vi "Initialize.vi"(7 "Serial Configuration":T1={"Baud Rate"=9600, "Parity"=0, "Data Bits"=8} {"Data Bits" items=["7"=7, "8"=8]; "Parity" items=["None", "Odd", "Even"]; "Baud Rate" items=["300"=300, "600"=600, "1200"=1200, "2400"=2400, "4800"=4800, "9600"=9600]}, 8 "error in (no error)":errorcluster, 9 "Reset (True)":bool=TRUE, 10 "ID Query (True)":bool=TRUE, 11 "VISA resource name":refnum<visa-resource-name>) -> (0 "error out":errorcluster, 3 "VISA resource name out":refnum<visa-resource-name>)   [LabVIEW 2022 SP3, in "Agilent 34420.lvlib"]
doc: "Establishes communication with the instrument and optionally performs an instrument identification query and/or an instrument reset. It also places the instrument in a default state needed for other instrument driver operations. Therefore, call this VI before calling other instrument driver VIs for this instrument. Generally, you need to call the Initialize VI only once at the beginning of an application."
uses:
  Agilent 34420.lvlib
  <vilib>/regexp/Match Regular Expression.xnode
  agilent_n6900_n7900_series/Agilent N6900 N7900 Series/Agilent N6900 N7900 Series.lvlib
panel:
  # "(c) 2008-2015 National Instruments Corp.  ALL RIGHTS RESERVED."
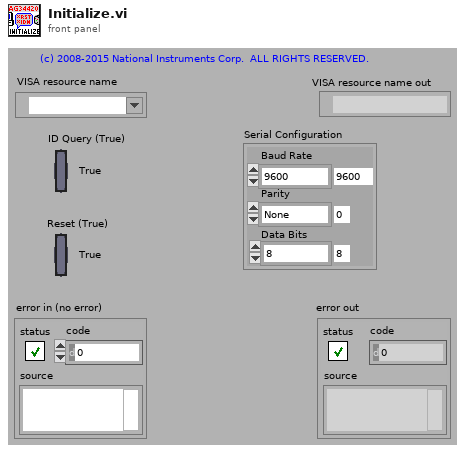
[diagram p1: front panel]
types:
  T1 = cluster{"Baud Rate":u32, "Parity":u16, "Data Bits":u16}
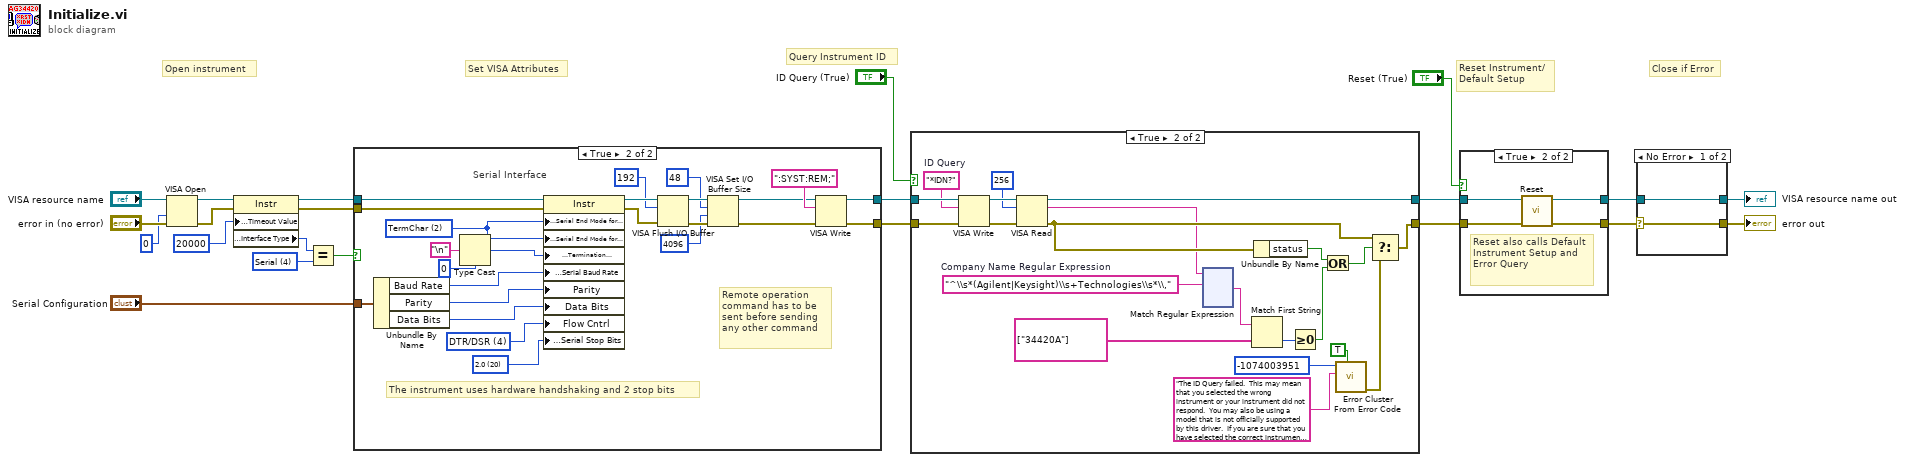
[diagram p0: block diagram]
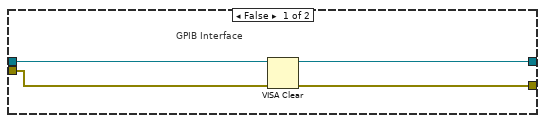
[diagram p2: hidden frame]
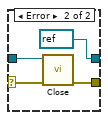
[diagram p3: hidden frame]
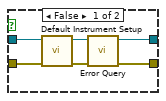
[diagram p4: hidden frame]
diagram:
  w11 = u16 4 items=["GPIB"=1, "VXI"=2, "GPIB-VXI"=3, "Serial"=4, "PXI"=5, "TCPIP"=6, "USB"=7] ("Interface Information:Interface Type")
  # "Set VISA Attributes"
  # "Close if Error"
  # "Query Instrument ID"
  # "Reset Instrument/\nDefault Setup"
  # "Open instrument"
  n1 = VISA Open(access mode=u32 0, error in (no error)="error in (no error)", VISA resource name="VISA resource name") -> (VISA resource name=w5:refnum<visa-resource-name>, error out=w4:errorcluster)  [unwired: 2 in]
  n2 = property class="Instr"(reference=w5, error in=w4, "General Settings:Timeout Value"=u32 20000) -> (reference out=w14:refnum<visa-resource-name>, error out=w13:errorcluster, "Interface Information:Interface Type"=w16:u16)
  n3 = Equal?(x=w16, y=w11) -> (x = y?=w12:bool)
  n4 = case shown="True" w12 {
    tunnel: [w24 w29] -> w2
    tunnel: [w23 w27] -> w1
    tunnel: w14 -> [w26 w49]
    tunnel: w13 -> [w25 w50]
    tunnel: "Serial Configuration" -> [_ w32]
    frame False {
      # "GPIB Interface"
      n5 = VISA Clear(VISA resource name=w26, error in (no error)=w25) -> (VISA resource name out=w24:refnum<visa-resource-name>, error out=w23:errorcluster)
    }
    frame True {
      w33 = u16 4 items=["None", "XON/XOFF", "RTS/CTS", "XON/XOFF & RTS/CTS", "DTR/DSR", "XON/XOFF & DTR/DSR"] ("Serial Settings:Flow Control")
      w36 = u16 20 items=["1.0"=10, "1.5"=15, "2.0"=20] ("Serial Settings:Stop Bits")
      w39 = u16 2 items=["None", "LastBit", "TermChar"] ("Serial Settings:Serial End Mode for Reads")
      # "Remote operation\ncommand has to be\nsent before sending\nany other command"
      # "The instrument uses hardware handshaking and 2 stop bits"
      # "Serial Interface"
      n6 = Unbundle By Name(w32) -> ("Baud Rate"=w37:u32, "Parity"=w35:u16, "Data Bits"=w34:u16)
      n7 = Type Cast(type=u8 0, x="\n" ("Line Feed Constant")) -> (*(type *) &x=w38:u8)
      n8 = property class="Instr"(reference=w49, error in=w50, "Serial Settings:Serial End Mode for Reads"=w39, "Serial Settings:Serial End Mode for Writes"=w39, "Message Based Settings:Termination Character"=w38, "Serial Settings:Serial Baud Rate"=w37, "Parity"=w35, "Data Bits"=w34, "Flow Cntrl"=w33, "Serial Settings:Serial Stop Bits"=w36) -> (reference out=w45:refnum<visa-resource-name>, error out=w47:errorcluster)
      n9 = VISA Flush I/O Buffer(VISA resource name=w45, mask (16)=u16 192, error in (no error)=w47) -> (VISA resource name out=w48:refnum<visa-resource-name>, error out=w46:errorcluster)
      n10 = VISA Set I/O Buffer Size(VISA resource name=w48, mask (16)=u16 48, size (4096)=u32 4096 ("size (0)"), error in (no error)=w46) -> (VISA resource name out=w30:refnum<visa-resource-name>, error out=w28:errorcluster)
      n11 = VISA Write(VISA resource name=w30, write buffer=":SYST:REM;", error in (no error)=w28) -> (VISA resource name out=w29:refnum<visa-resource-name>, error out=w27:errorcluster)  [unwired: 1 out]
    }
  }
  n12 = case shown="True" "ID Query (True)" {
    tunnel: [w51 w73] -> w21
    tunnel: [w52 w70] -> w22
    tunnel: w2 -> [w52 w71]
    tunnel: w1 -> [w51 w72]
    frame False {
    }
    frame True {
      w53 = "^\\s*(Agilent|Keysight)\\s+Technologies\\s*\\,"  # Company Name Regular Expression
      w66 = "*IDN?"  # ID Query
      n13 = VISA Write(VISA resource name=w71, write buffer=w66, error in (no error)=w72) -> (VISA resource name out=w69:refnum<visa-resource-name>, error out=w68:errorcluster)  [unwired: 1 out]
      n14 = VISA Read(VISA resource name=w69, byte count=u32 256, error in (no error)=w68) -> (VISA resource name out=w70:refnum<visa-resource-name>, read buffer=w55:string, error out=w61:errorcluster)  [unwired: 1 out]
      n15 = xnode "Match Regular Expression"("input string"=w55, "regular expression"=w53) -> ("after match"=w54:string)  [unwired: 4 in, 4 out]
      n16 = Match First String(2:string[] ["34420A"] ("string array"), 3:w54) -> (0:w57:i32)  [unwired: 1 out]
      n17 = Unbundle By Name(w61) -> ("status"=w60:bool)
      n18 = Greater Or Equal To 0?(x=w57) -> (x >= 0?=w59:bool)
      n19 = Or(x=w60, y=w59) -> (x .or. y?=w58:bool)
      n20 = call <vilib>:"Error Cluster From Error Code.vi"("show call chain? (False)"=TRUE, "error message (\"\")"="The ID Query failed.  This may mean that you selected the wrong instrument or your instrument did not respond.  You may also be using a model that is not officially supported by this driver.  If you are sure that you have selected the correct instrument and it is responding, try disabling the ID Query." ("Source (VI Name)"), "error code (0)"=-1074003951 ("Code")) -> ("error out"=w65:errorcluster)  [unwired: 6 in]
      n21 = Select(t=w61, s=w58, f=w65) -> (s? t:f=w73:errorcluster)
    }
  }
  n22 = case shown="True" "Reset (True)" {
    tunnel: w21 -> [w195 w199]
    tunnel: [w192 w197] -> w6
    tunnel: w22 -> [w196 w200]
    tunnel: [w193 w198] -> w7
    frame False {
      n23 = call "Default Instrument Setup.vi"("error in (no error)"=w195, "VISA resource name"=w196) -> ("error out"=w191:errorcluster, "VISA resource name out"=w194:refnum<visa-resource-name>)  [unwired: 8 in]
      n24 = call "Error Query.vi"("error in (no error)"=w191, "VISA resource name"=w194) -> ("error out"=w192:errorcluster, "VISA resource name out"=w193:refnum<visa-resource-name>)  [unwired: 6 in, 2 out]
    }
    frame True {
      # "Reset also calls Default Instrument Setup and Error Query"
      n25 = call "Reset.vi"("error in (no error)"=w199, "VISA resource name"=w200) -> ("error out"=w197:errorcluster, "VISA resource name out"=w198:refnum<visa-resource-name>)  [unwired: 8 in]
    }
  }
  n26 = case shown="No Error" w6 {
    selector: w6 -> [w201 w204]
    tunnel: w7 -> [w202 w205]
    tunnel: [w202 refnum<visa-resource-name> refnum ("VISA resource name out")] -> w9
    tunnel: [w201 w206] -> w8
    frame No Error {
    }
    frame Error {
      n27 = call "Close.vi"("error in (no error)"=w204, "VISA resource name"=w205) -> ("error out"=w206:errorcluster)  [unwired: 9 in]
    }
  }
  "VISA resource name out" <- w9
  "error out" <- w8
